vi "DiscArchiver.check free disc fraction.vi"(0 "i ref in":refnum<vi>, 3 "ms timeout (10000)":i32=10000, 5 "error in (no error)":errorcluster) -> (14 "i ref out":refnum<vi>, 16 "disc size alarm":bool, 17 "timed out":bool, 19 "error out":errorcluster)   [LabVIEW 2014, in "DiscArchiver.lvlib"]
doc: "Checks, if the faction of available disk size is below the alarm level. If yes, the error will be returned in error out."
uses:
  DiscArchiver.lvlib
  CS_Core/CSSystem/CoreDefs/CoreDefs.error_type.ctl
  CS_Core/CSSystem/CoreLib/CoreLib.lvlib
  CSlibraries/UtilityLib/UtilityLib.lvlib
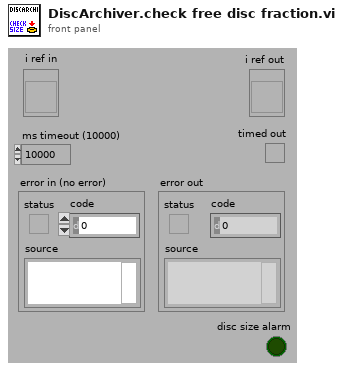
[diagram p1: front panel]
types:
  T1 = typedef "CoreDefs.error_type.ctl" = enum16{"no error", "can't load process", "can't unload process", "process does not exist", "can't install process", "can't remove process", "unknown function", "time out", "can't execute function", "duplicate queue name", "super not found", "caller queue invalid", "can't ping process", "unknown error", "VISA Error", "VISA timeout", "GPIB timeout", "GPIB error", "communication error", "data type mismatch", "can't read data from OPC server", "can't write data to OPC server", "OET error", "function not implemented", "process already exists", "invalid Shared Variable name", "error writing Shared Variable", "error reading Shared Variable", "invalid client name", "corrupt database", "unknown class", "call not authorized", "parameter out of range", "OET timeout: can't get data to modify", "invalid queue name", "requested operation incompatible with current state", "event undefined", "event disabled", "state undefined", "caller is not a friend", "EventBuilder: bad eventID", "EventBuilder: no DAQ devices", "a thread must not stop itself", "UNUSED ELEMENT4", "DiscArchiver: eventData incomplete", "DiscArchiver: eventData does not belong to run", "DiscArchiver: can't open file", "DiscArchiver: can't write to file", "DiscArchiver: available disc space low", "can't acquire semaphore", "error reading data from database", "notifier object is not existing", "can't register process", "can't unregister process", "illegal event type", "object disabled", "object already exists", "can't change state", "Instrument not found", "no connection to remote node", "invalid reference", "N/A", "UNUSED ELEMENT 1", "element not found", "illegal TCP/IP connection detected", "object does not exist", "invalid access ID", "unknown CS system", "invalid privilige", "unsupported data type", "unsupported server type", "IO server already exists", "Shared Variable already exists"}
  T2 = typedef "DiscArchiver.lvlib/DiscArchiver.i attribute.ctl" = cluster{"file prefix":string, "actual file":string, "nOfEvents":i32, "file":refnum<file>, "eventBuilder":string, "disc size alarm":bool, "dataDescription":string, "dataDescriptionURL":string, "eventDataURL":string, "headerID":dbl, "completeData":bool, "nOfEventsID":i32, "dataFileID":i32}
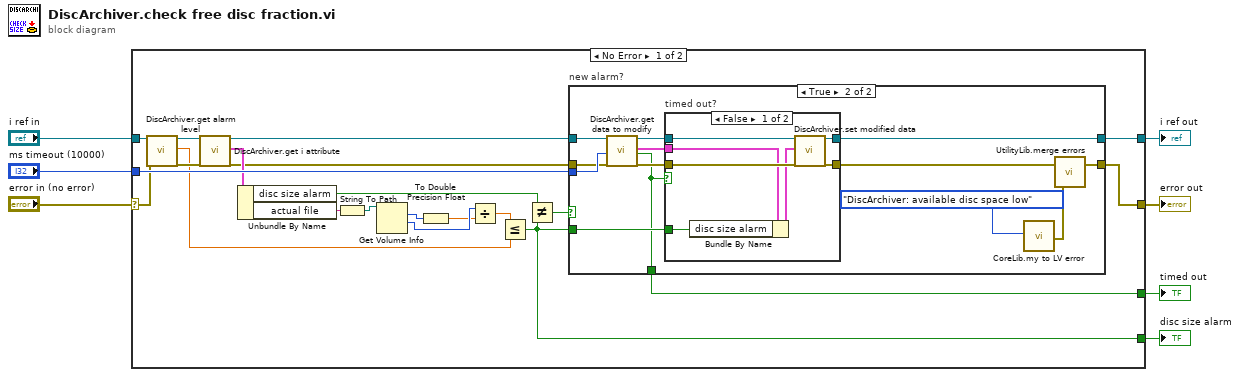
[diagram p0: block diagram]
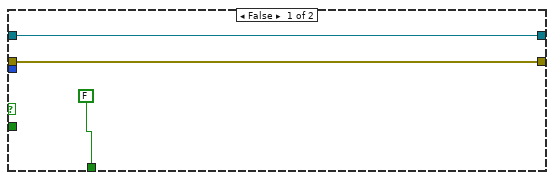
[diagram p2: hidden frame]
diagram:
  n1 = case shown="No Error" "error in (no error)" {
    selector: "error in (no error)" -> [w9 w54]
    tunnel: [w28 w55] -> w7
    tunnel: "ms timeout (10000)" -> [w27 _]
    tunnel: "i ref in" -> [w26 w55]
    tunnel: [w14 _] -> w4
    tunnel: [w11 _] -> w3
    tunnel: [w10 w54] -> w2
    frame No Error {
      n2 = call "DiscArchiver.get alarm level.vi"("i ref in"=w26, "error in (no error)"=w9) -> ("i ref out"=w25:refnum<vi>, "alarm level"=w17:dbl, "error out"=w24:errorcluster)  [unwired: 15 in]
      n3 = call "DiscArchiver.get i attribute.vi"("i ref in"=w25, "error in (no error)"=w24) -> ("i ref out"=w12:refnum<vi>, "i attribute"=w23:T2, "error out"=w13:errorcluster)  [unwired: 15 in]
      n4 = Unbundle By Name(w23) -> ("disc size alarm"=w16:bool, "actual file"=w22:string)
      n5 = String To Path(string=w22) -> (path=w21:path)
      n6 = Get Volume Info(11:w21) -> (1:w20:i64, 2:w8:i64)  [unwired: 1 in, 4 out]
      n7 = To Double Precision Float(number=w8) -> (double precision float=w19:dbl)
      n8 = Divide(x=w20, y=w19) -> (x/y=w18:dbl)
      n9 = Less Or Equal?(x=w18, y=w17) -> (x <= y?=w14:bool)
      n10 = Not Equal?(x=w16, y=w14) -> (x != y?=w15:bool)
      n11 = case "new alarm?" shown="True" w15 {
        tunnel: [w29 w44] -> w28
        tunnel: w27 -> [_ w40]
        tunnel: w14 -> [_ w39]
        tunnel: w13 -> [w30 w38]
        tunnel: w12 -> [w29 w37]
        tunnel: [FALSE ("timed out") w35] -> w11
        tunnel: [w30 w34] -> w10
        frame False {
        }
        frame True {
          n12 = call "DiscArchiver.get data to modify.vi"("i ref in"=w37, "ms timeout (10000)"=w40, "error in (no error)"=w38) -> ("i ref out"=w43:refnum<vi>, "i attribute"=w41:T2, "timed out"=w35:bool, "error out"=w42:errorcluster)  [unwired: 13 in]
          n13 = case "timed out?" shown="False" w35 {
            tunnel: [w51 w52] -> w33
            tunnel: [w50 w53] -> w44
            tunnel: w43 -> [w49 w53]
            tunnel: w42 -> [w48 w52]
            tunnel: w41 -> [w46 _]
            tunnel: w39 -> [w45 _]
            frame False {
              n14 = Bundle By Name(cluster=w46, "disc size alarm"=w45) -> (w47:T2)
              n15 = call "DiscArchiver.set modified data.vi"("i ref in"=w49, "i attribute"=w47, "error in (no error)"=w48) -> ("i ref out"=w50:refnum<vi>, "error out"=w51:errorcluster)  [unwired: 15 in]
            }
            frame True {
            }
          }
          n16 = call "CoreLib.my to LV error.vi"("ErrorTypes"=CoreDefs.error_type."DiscArchiver: available disc space low") -> ("myErrorCluster"=w32:errorcluster)  [unwired: 17 in, 1 out]
          n17 = call "UtilityLib.merge errors.vi"("error2 (no error)"=w32, "error1 (no error)"=w33) -> ("error out"=w34:errorcluster)
        }
      }
    }
    frame Error {
    }
  }
  "error out" <- w2
  "i ref out" <- w7
  "timed out" <- w3
  "disc size alarm" <- w4
